vi "Servo-Motor_Api.vi"(7 "角度":dbl, 8 "Error In":errorcluster, 11 "伺服馬達角位":tag="A/PWM0") -> (0 "Error Out":errorcluster)   [LabVIEW 2019]
uses:
  <vilib>/myRIO/Instrument Drivers/Onboard IO/PWM/PWM.lvlib
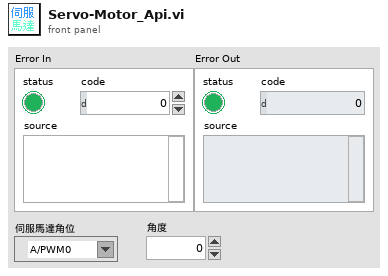
[diagram p1: front panel]
types:
  T1 = typedef "PWM.lvlib/PWM Reference.ctl" = cluster{"myRIO Reference":T2, "PWM Channels Enum":T6, "PWM Configuration":T7}
  T2 = typedef "myRIO Generic Hardware Reference.ctl" = cluster{"myRIO Model":T3, "myRIO Hardware Reference":T4}
  T3 = typedef "Hardware Version Enum.ctl" = enum16{"Unknown", "myRIO-1900", "myRIO-1950", "roboRIO", "NI ELVIS RIO CM", "ELVIS III"}
  T4 = typedef "myRIO v1.0 Reference.ctl" = cluster{"Generic FPGA Reference":T5, "Allow multiple opens":bool}
  T5 = typedef "Generic FPGA Reference.ctl" = refnum<k20>
  T6 = typedef "PWM Channels Enum.ctl" = enum16{"Not Connected", "C/PWM0", "C/PWM1", "A/PWM0", "A/PWM1", "A/PWM2", "A/PWM3", "A/PWM4", "A/PWM5", "A/PWM6", "A/PWM7", "A/PWM8", "A/PWM9", "A/PWM10", "A/PWM11", "A/PWM12", "A/PWM13", "A/PWM14", "A/PWM15", "A/PWM16", "A/PWM17", "A/PWM18", "A/PWM19", "B/PWM0", "B/PWM1", "B/PWM2", "B/PWM3", "B/PWM4", "B/PWM5", "B/PWM6", "B/PWM7", "B/PWM8", "B/PWM9", "B/PWM10", "B/PWM11", "B/PWM12", "B/PWM13", "B/PWM14", "B/PWM15", "B/PWM16", "B/PWM17", "B/PWM18", "B/PWM19", "PWM/PWM0", "PWM/PWM1", "PWM/PWM2", "PWM/PWM3", "PWM/PWM4", "PWM/PWM5", "PWM/PWM6", "PWM/PWM7", "PWM/PWM8", "PWM/PWM9"}
  T7 = typedef "PWM.lvlib/PWM Configuration.ctl" = cluster{"Frequency":dbl, "Duty Cycle":dbl}
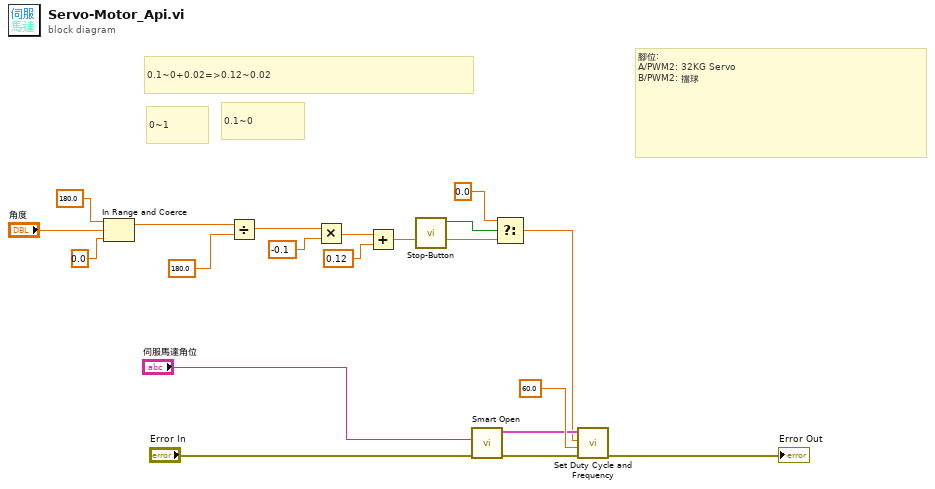
[diagram p0: block diagram]
diagram:
  # "腳位:\nA/PWM2: 32KG Servo\nB/PWM2: 擋球"
  # "0.1~0+0.02=>0.12~0.02"
  # "0.1~0"
  # "0~1"
  n1 = In Range and Coerce(upper limit=180.0, x="角度", lower limit=0.0) -> (coerced(x)=w10:dbl)  [unwired: 1 out]
  n2 = Divide(x=w10, y=180.0) -> (x/y=w8:dbl)
  n3 = Multiply(x=w8, y=-0.1) -> (x*y=w6:dbl)
  n4 = Add(x=w6, y=0.12) -> (x+y=w4:dbl)
  n5 = call "Stop-Button.vi"() -> ("顯示按下?"=w2:bool)  [unwired: 10 in, 1 out]
  n6 = call <vilib>:"Smart Open.vi"("error in (no error)"="Error In", "Channel Name"="伺服馬達角位") -> ("error out"=w16:errorcluster, "PWM Ref Out"=w17:T1)  [unwired: 8 in]
  n7 = Select(t=0.0, s=w2, f=w4) -> (s? t:f=w1:dbl)
  n8 = call <vilib>:"Set Duty Cycle and Frequency.vi"("error in (no error)"=w16, "Frequency [Hz]"=60.0, "Duty Cycle"=w1, "PWM Ref In"=w17) -> ("error out"=→"Error Out":errorcluster)  [unwired: 5 in, 1 out]
